vi "Stimulus Waveform.vi"() -> ()   [LabVIEW 2010]
doc: "I. Description:\nThis example demonstrates how to output a continuous periodic waveform using an internal sample clock.\n\nII. Instructions for Running:\n1. Select the Physical Channel to correspond to where your signal is output on the DAQ device.\n2. Enter the Minimum and Maximum Voltage Ranges\n3. Specify the Desired Frequency of the output Waveform\n4. Enter the Waveform Information. See the documentation of the Waveform Buffer Generation SubVI for information on each parameter.\n\nIII. Block Diagram Steps:\n1. Create an Analog Output Voltage channel.\n2. Call the DAQmx Timing (Use Waveform) VI which sets the sample clock rate based on the input waveform parameters, and set the sample mode to Continuous.\n3. Write the waveform to the output buffer.\n4. Call the Start VI.\n5. Loop continuously until the user presses the Stop button. Check for errors every 100 ms using the Is Task Done? VI\n6. Clear the Task\n7. Use the popup dialog box to display an error or warning if any.\n\nIV. I/O Connections Overview:\nMake sure your signal output terminal matches the Physical Channel I/O Control. For further connection information, refer to your hardware reference manual."
uses:
  <vilib>/Utility/error.llb/DialogType.ctl
  <vilib>/DAQmx/write.llb/DAQmx Write (Analog 1D Wfm NChan NSamp).vi
  <vilib>/DAQmx/create/channels.llb/DAQmx Create Channel (AO-Voltage-Basic).vi
  <vilib>/DAQmx/configure/timing.llb/DAQmx Timing (Use Waveform).vi
  <vilib>/daqmx/miscellaneous.llb/DAQmx Fill In Error Info.vi
panel:
  out "Resulting Frequency":dbl=1000.0 format="%.2f"
  in  "Cycles per Buffer":i32=15
  in  "Waveform Type":T1(ring)
  in  "Desired Frequency":dbl=10000.0 format="%.2f"
  in  "Samples per Buffer":dbl=750.0
  in  "Amplitude":dbl=1.0 format="%0.2p"
  out "Waveform Graph":waveform(dbl)[](graph)=[{"t0"=timestamp(0 s since 1904-01-01), "dt"=2e-05, "Y"=array[250 elements]}, {"t0"=timestamp(0.005 s since 1904-01-01), "dt"=2e-05, "Y"=array[250 elements]}] caption="Output Waveform"
  in  "Physical Channels":tag="PXI1Slot3/ao0"
  in  "Minimum Value":dbl=-10.0 format="%0.2f"
  in  "Maximum Value":dbl=10.0 format="%0.2f"
  in  "stop":bool
  # "For instructions, select Help>>Show Context Help"
  # "Channel Parameters"
  # "Timing Parameters"
  # "Waveform Information"
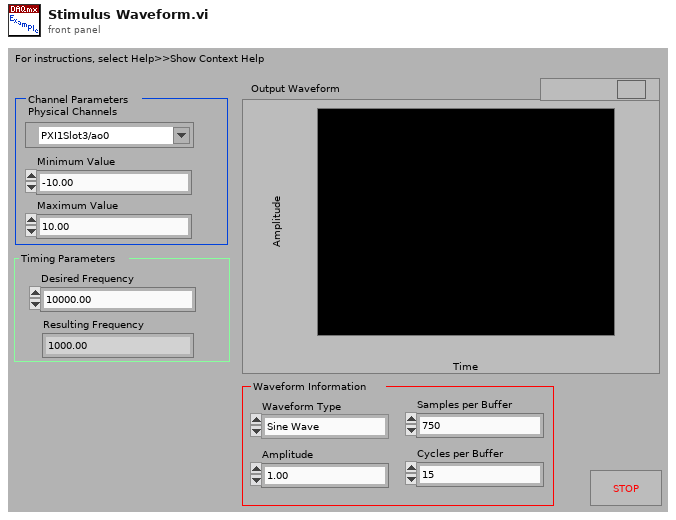
[diagram p1: front panel]
types:
  T1 = enum16{"Sine Wave", "Triangle Wave", "Square Wave", "Sawtooth Wave"}
  T2 = typedef "DialogType.ctl" = u16
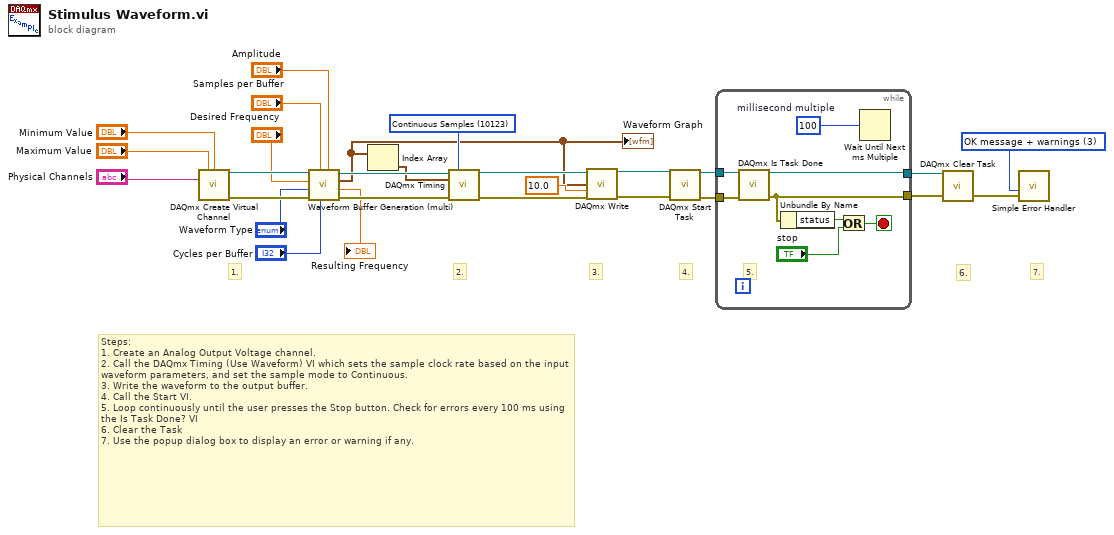
[diagram p0: block diagram]
diagram:
  w15 = T2 3 items=["no dialog", "OK message", "continue or stop message", "OK message + warnings", "continue/stop + warnings"] ("type of dialog (OK msg:1)")
  w26 = 10123 items=["Finite Samples"=10178, "Continuous Samples"=10123] ("sample mode")
  # "7."
  # "6."
  # "Steps: \n1. Create an Analog Output Voltage channel.\n2. Call the DAQmx Timing (Use Waveform) VI which sets the sample clock rate based on the input waveform parameters, and set the sample mode to Continuous.\n3. Write the waveform to the output buffer.\n4. Call the Start VI.\n5. Loop continuously until the user presses the Stop button. Check for errors every 100 ms using the Is Task Done? VI\n6. Clear the Task\n7. Use the popup dialog box to display an error or warning if any."
  # "4."
  # "3."
  # "2."
  # "1."
  n1 = call-poly <vilib>:"DAQmx Create Virtual Channel.vi"("maximum value"="Maximum Value", "minimum value"="Minimum Value", "physical channels"="Physical Channels") -> ("task out"=w10:refnum<k21>, "error out"=w9:errorcluster)  [unwired: 11 in]
  n2 = call "Waveform Buffer Generation (multi).vi"("Amplitude"="Amplitude", "Cycles per Buffer"="Cycles per Buffer", "Samples per Buffer"="Samples per Buffer", "error in (no error)"=w9, "Waveform Type"="Waveform Type", "Desired Frequency"="Desired Frequency", "task/channels in"=w10) -> ("error out"=w11:errorcluster, "Resulting Frequency"=→"Resulting Frequency":dbl, "Waveform"=w2:waveform(dbl)[], "task out"=w12:refnum<k21>)  [unwired: 1 out]
  "Waveform Graph" <- w2
  n3 = Index Array(array=w2) -> (element=w1:waveform(dbl))  [unwired: 1 in]
  n4 = call-poly <vilib>:"DAQmx Timing.vi"("task/channels in"=w12, "sample mode"=w26, "waveform"=w1, "error in"=w11) -> ("task out"=w18:refnum<k21>, "error out"=w17:errorcluster)  [unwired: 10 in]
  n5 = call-poly <vilib>:"DAQmx Write.vi"("task/channels in"=w18, "data"=w2, "timeout"=10.0 ("Wirite Timeout"), "error in"=w17) -> ("task out"=w23:refnum<k21>, "error out"=w22:errorcluster)  [unwired: 9 in, 1 out]
  n6 = call <vilib>:"DAQmx Start Task.vi"("task/channels in"=w23, "error in"=w22) -> ("task out"=w16:refnum<k21>, "error out"=w20:errorcluster)  [unwired: 12 in]
  n7 = while {
    tunnel: w16 -> [w35]
    tunnel: [w34] -> w14
    tunnel: w20 -> [w33]
    tunnel: [w32] -> w13
    stop <- w30 stop-if-true
    w31 = u32 100  # millisecond multiple
    # "5."
    n8 = call <vilib>:"DAQmx Is Task Done.vi"("task/channels in"=w35, "error in"=w33) -> ("task out"=w34:refnum<k21>, "error out"=w32:errorcluster)  [unwired: 11 in, 1 out]
    n9 = Unbundle By Name(w32) -> ("status"=w29:bool)
    n10 = Or(x=w29, y="stop") -> (x .or. y?=w30:bool)
    n11 = Wait Until Next ms Multiple(millisecond multiple=w31) -> ()  [unwired: 1 out]
  }
  n12 = call <vilib>:"DAQmx Clear Task.vi"("task in"=w14, "error in"=w13) -> ("error out"=w27:errorcluster)  [unwired: 13 in]
  n13 = call <vilib>:"Simple Error Handler.vi"("type of dialog (OK msg:1)"=w15, "error in (no error)"=w27) -> ()  [unwired: 3 in, 5 out]
